vi "OtwieranieCMDPrzez Labwiew.vi"() -> ()   [LabVIEW 2015]
uses:
  <vilib>/Utility/NIReport.llb/Append Report Text (str wrap).vi
  <vilib>/Utility/NIReport.llb/NI_report.lvclass
panel:
  in  "text options":T1
  in  "font settings":T2={"Charset (-1)"=-1, "Weight (-1)"=-1, "Name"="", "Size"=" "}
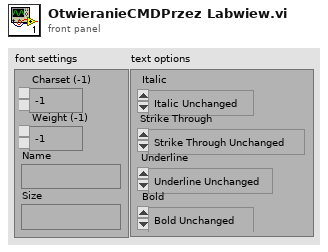
[diagram p1: front panel]
types:
  T1 = cluster{"Italic":enum16{"Italic Unchanged", "Italic On", "Italic Off"}, "Strike Through":enum16{"Strike Through Unchanged", "Strike Through On", "Strike Through Off"}, "Underline":enum16{"Underline Unchanged", "Underline On", "Underline Off"}, "Bold":enum16{"Bold Unchanged", "Bold On", "Bold Off"}}
  T2 = cluster{"Charset (-1)":i16, "Weight (-1)":i16, "Name":string, "Size":string}
  T3 = enum16{"Standard Report", "HTML", "Word", "Excel"}
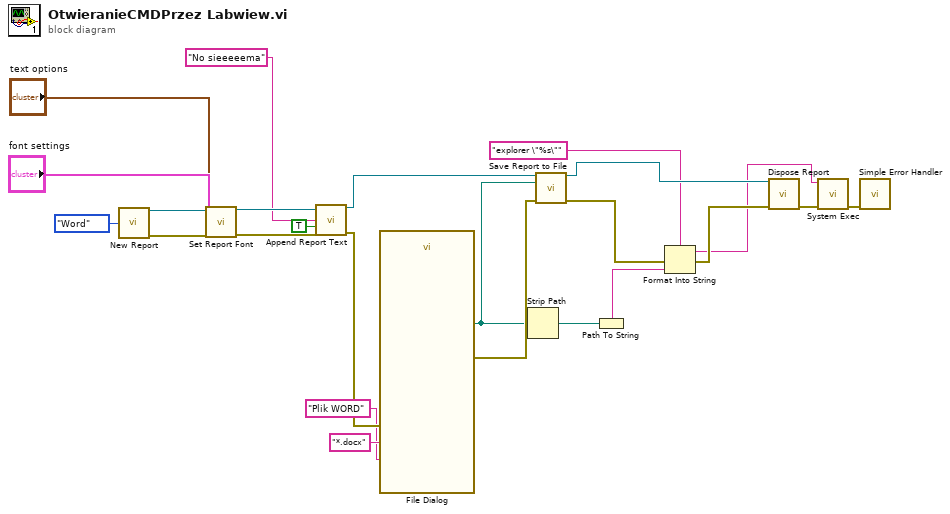
[diagram p0: block diagram]
diagram:
  n1 = call <vilib>:"New Report.vi"("report type"=T3."Word") -> ("report out"=w23:refnum<class "NI_report.lvclass">, "error out"=w19:errorcluster)  [unwired: 13 in]
  n2 = call-dynamic "Set Report Font.vi"("report in"=w23, "text options"="text options", "font settings"="font settings", "error in (no error)"=w19) -> ("report out"=w22:refnum<class "NI_report.lvclass">, "error out"=w18:errorcluster)  [unwired: 9 in, 1 out]
  n3 = call-poly <vilib>:"Append Report Text.vi"("report in"=w22, "text"="No sieeeeema", "append on new line? (F)"=TRUE, "error in (no error)"=w18) -> ("report out"=w21:refnum<class "NI_report.lvclass">, "error out"=w17:errorcluster)  [unwired: 8 in, 2 out]
  n4 = call "File Dialog"("error in"=w17, "pattern (all files)"="*.docx", "pattern label"="Plik WORD" ("default name")) -> ("selected path"=w9:path, "error out"=w16:errorcluster)  [unwired: 9 in, 2 out]
  n5 = Strip Path(path=w9) -> (stripped path=w1:path)  [unwired: 1 out]
  n6 = call-dynamic "Save Report to File.vi"("report in"=w21, "report file path"=w9, "error in (no error)"=w16) -> ("report out"=w20:refnum<class "NI_report.lvclass">, "error out"=w8:errorcluster)  [unwired: 11 in]
  n7 = Path To String(path=w1) -> (string=w4:string)
  n8 = Format Into String(format string="explorer \"%s\"", error in=w8, w4) -> (resulting string=w3:string, error out=w7:errorcluster)  [unwired: 1 in]
  n9 = call-dynamic "Dispose Report.vi"("report in"=w20, "error in (no error)"=w7) -> ("error out"=w6:errorcluster)  [unwired: 13 in]
  n10 = call <vilib>:"System Exec.vi"("error in (no error)"=w6, "command line"=w3) -> ("error out"=w5:errorcluster)  [unwired: 6 in, 3 out]
  n11 = call <vilib>:"Simple Error Handler.vi"("error in (no error)"=w5) -> ()  [unwired: 4 in, 5 out]
